vi "Edit Item.vi"(3 "Error in":errorcluster, 5 "Item":u32) -> (0 "Error out":errorcluster)   [LabVIEW 2020]
uses:
  <vilib>/Utility/config.llb/Write Key (String).vi
  <vilib>/Utility/config.llb/NI_LVConfig.lvlib
panel:
  in  "Description":string
  in  "Access Level":enum16{"read-only", "write-only", "read/write"}(ring)
  in  "Data Type":enum16{"Double"}(ring)
  in  "Name":string
  in  "Cancel Button":bool
  in  "OK Button":bool
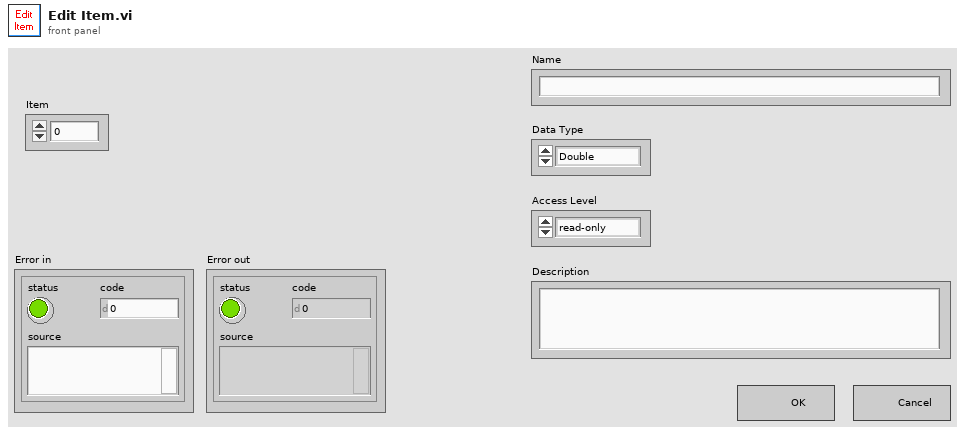
[diagram p1: front panel]
types:
  T1 = cluster{"Name":string, "Data type":u16, "Access level":u16, "Description":string}[]
  T2 = cluster{"Name":string, "Data type":u16, "Access level":u16, "Description":string}
  T3 = typedef "NI_LVConfig.lvlib/Config Data RefNum.ctl" = refnum<k1>
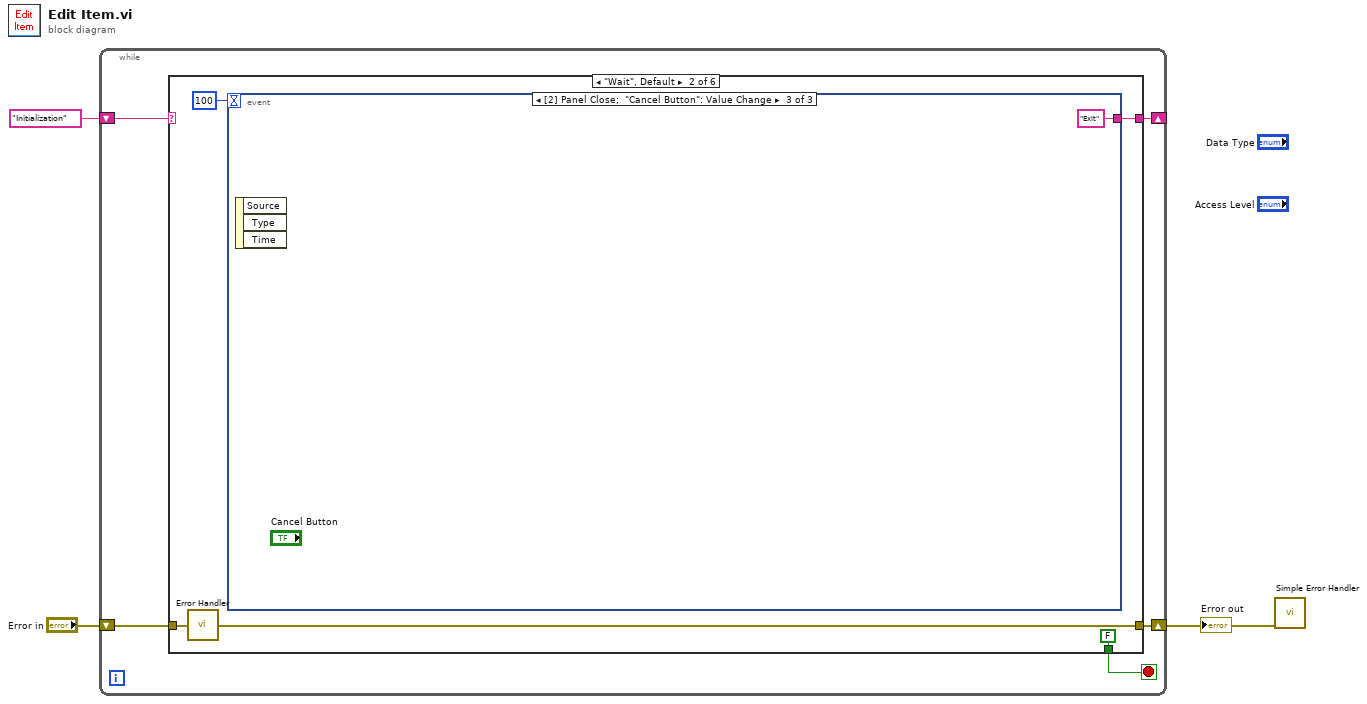
[diagram p0: block diagram]
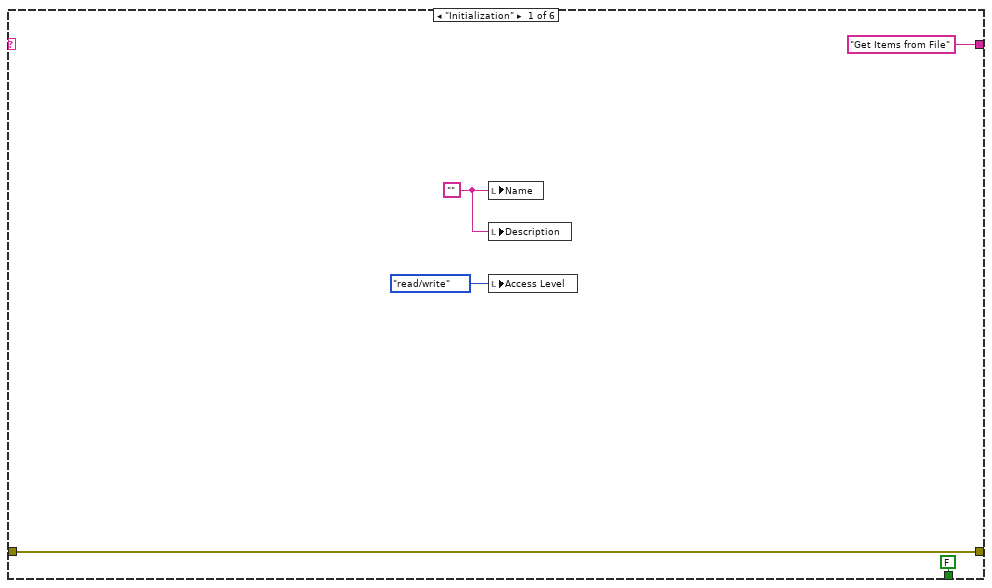
[diagram p2: hidden frame]
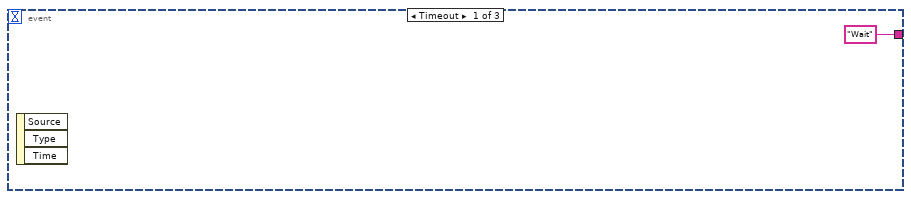
[diagram p3: hidden frame]
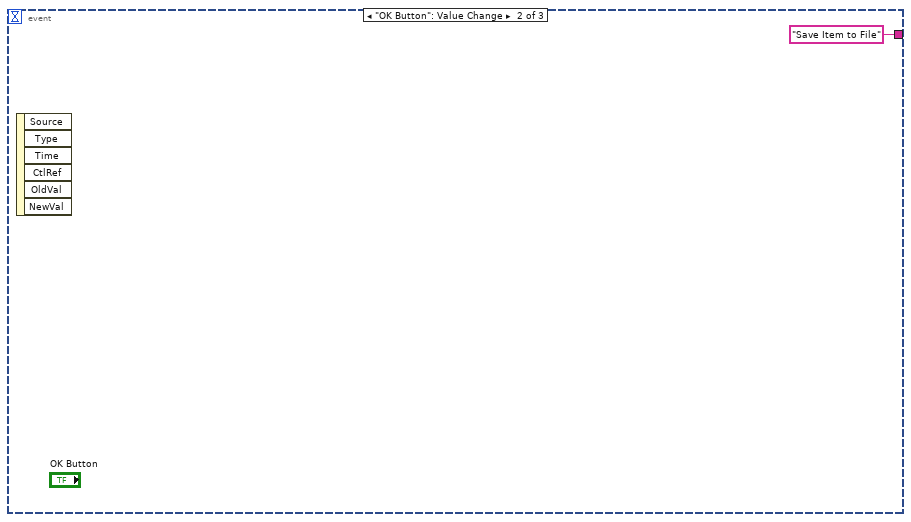
[diagram p4: hidden frame]
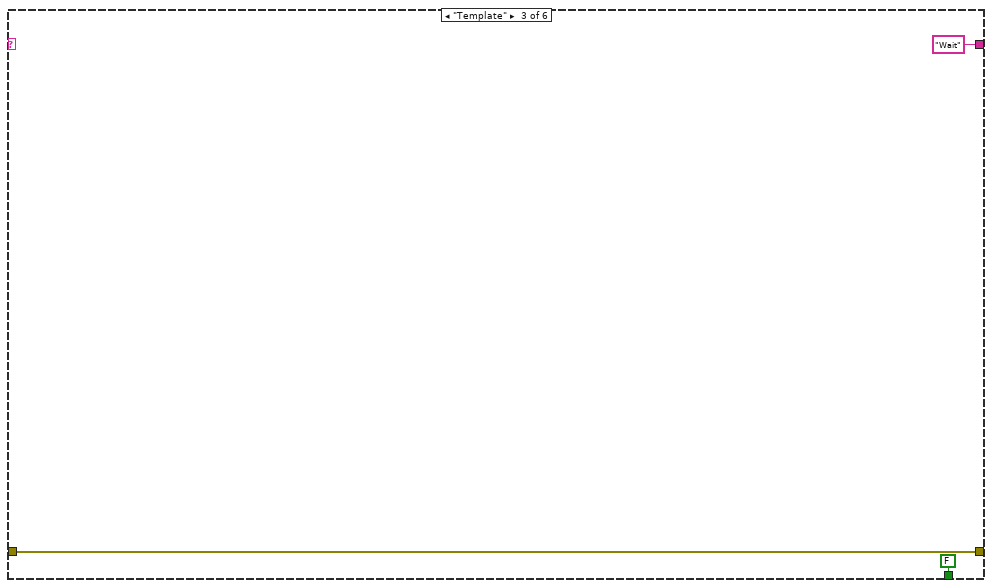
[diagram p5: hidden frame]
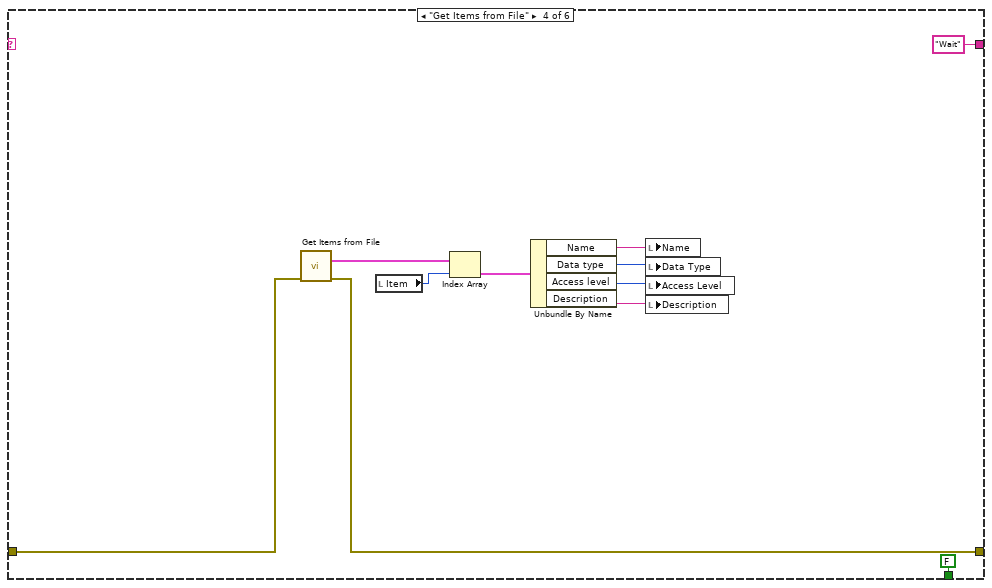
[diagram p6: hidden frame]
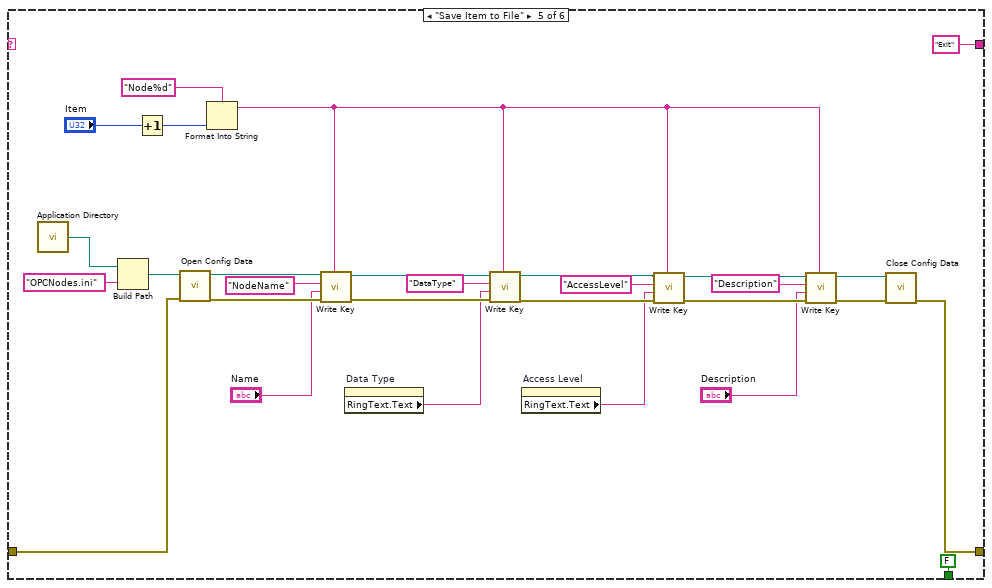
[diagram p7: hidden frame]
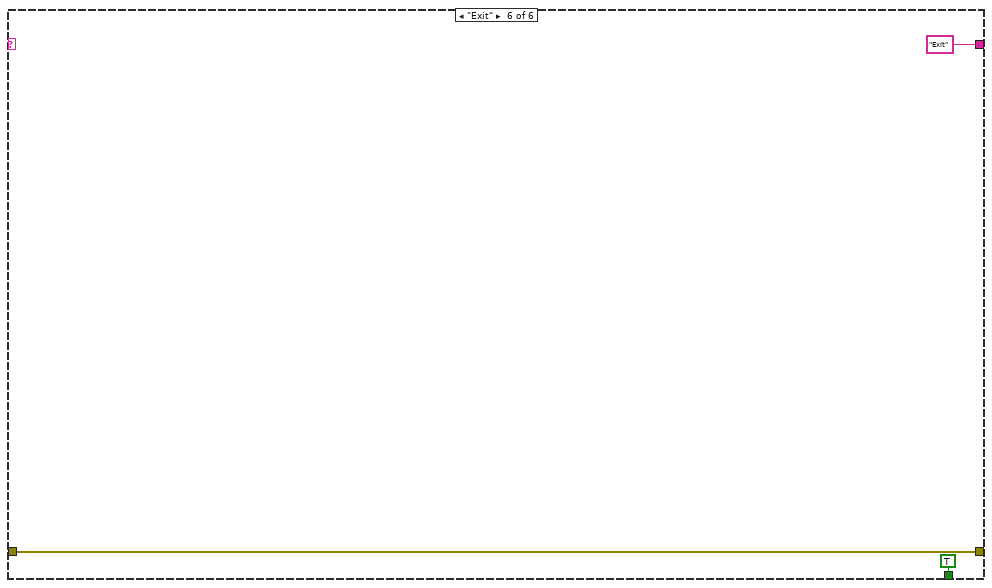
[diagram p8: hidden frame]
diagram:
  n1 = while {
    shift-right: [w7] -> _
    shift-left: "Initialization" -> [w8]
    shift-right: [w4] -> w1
    shift-left: "Error in" -> [w5]
    stop <- w6 stop-if-true
    n2 = case shown="\"Wait\", Default" w8 {
      tunnel: ["Get Items from File" w16 "Wait" "Wait" "Exit" "Exit"] -> w7
      tunnel: [FALSE FALSE FALSE FALSE FALSE TRUE] -> w6
      tunnel: w5 -> [w11 w14 w22 w25 w44 w65]
      tunnel: [w11 w15 w22 w26 w40 w65] -> w4
      frame "Initialization" {
        w9 = ""
        n3 = local write "Name"(w9) -> ()
        n4 = local write "Description"(w9) -> ()
        n5 = local write "Access Level"(enum16{"read-only", "write-only", "read/write"}."read/write" ("Access Level")) -> ()
      }
      frame "Wait", Default {
        n6 = call "Error Handler.vi"("Error in"=w14) -> ("Error out"=w15:errorcluster)
        n7 = event shown="[2] Panel Close;  \"Cancel Button\": Value Change" {
          selector: _ -> [_ _ _]
          dyn-events: _ -> [_ _ _]
          timeout: 100 ("ms") -> [_ _ _]
          tunnel: ["Wait" "Save Item to File" "Exit"] -> w16
          event Timeout {
            n8 = event-data() -> ()  [unwired: 1 in, 3 out]
          }
          event "OK Button": Value Change {
            n9 = event-data() -> ()  [unwired: 1 in, 6 out]
          }
          event Panel Close; "Cancel Button": Value Change {
            n10 = event-data() -> ()  [unwired: 1 in, 3 out]
          }
        }
      }
      frame "Template" {
      }
      frame "Get Items from File" {
        n11 = call "Get Items from File.vi"("Error in"=w25) -> ("Error out"=w26:errorcluster, "Items"=w33:T1)  [unwired: 9 in]
        n12 = local read "Item"() -> (w32:u32)
        n13 = Index Array "Index Array"(array=w33, index=w32) -> (element=w31:T2)
        n14 = Unbundle By Name(w31) -> ("Name"=w30:string, "Data type"=w29:u16, "Access level"=w28:u16, "Description"=w27:string)
        n15 = local write "Name"(w30) -> ()
        n16 = local write "Data Type"(w29) -> ()
        n17 = local write "Access Level"(w28) -> ()
        n18 = local write "Description"(w27) -> ()
      }
      frame "Save Item to File" {
        n19 = call <vilib>:"Application Directory.vi"() -> ("Application Directory"=w62:path)
        n20 = Build Path(base path=w62, name or relative path="OPCNodes.ini") -> (appended path=w60:path)
        n21 = Increment(x="Item") -> (x+1=w37:u32)
        n22 = call <vilib>:"Open Config Data.vi"("error in (no error)"=w44, "configuration file path"=w60) -> ("error out"=w54:errorcluster, "refnum"=w59:T3)  [unwired: 7 in, 1 out]
        n23 = Format Into String(format string="Node%d" ("section"), w37) -> (resulting string=w36:string)  [unwired: 2 in, 1 out]
        n24 = call-poly <vilib>:"Write Key.vi"("section"=w36, "error in (no error)"=w54, "value"="Name", "key"="NodeName", "refnum"=w59) -> ("error out"=w53:errorcluster, "refnum out"=w47:T3)  [unwired: 4 in, 1 out]
        n25 = property on="Data Type" class="Enum (strict)"() -> ("RingText.Text"=w49:string)  [unwired: 2 in, 2 out]
        n26 = call-poly <vilib>:"Write Key.vi"("section"=w36, "error in (no error)"=w53, "value"=w49, "key"="DataType", "refnum"=w47) -> ("error out"=w52:errorcluster, "refnum out"=w46:T3)  [unwired: 4 in, 1 out]
        n27 = property on="Access Level" class="Enum (strict)"() -> ("RingText.Text"=w48:string)  [unwired: 2 in, 2 out]
        n28 = call-poly <vilib>:"Write Key.vi"("section"=w36, "error in (no error)"=w52, "value"=w48, "key"="AccessLevel", "refnum"=w46) -> ("error out"=w51:errorcluster, "refnum out"=w45:T3)  [unwired: 4 in, 1 out]
        n29 = call-poly <vilib>:"Write Key.vi"("section"=w36, "error in (no error)"=w51, "value"="Description", "key"="Description", "refnum"=w45) -> ("error out"=w41:errorcluster, "refnum out"=w42:T3)  [unwired: 4 in, 1 out]
        n30 = call <vilib>:"Close Config Data.vi"("error in (no error)"=w41, "refnum"=w42) -> ("error out"=w40:errorcluster)  [unwired: 8 in, 1 out]
      }
      frame "Exit" {
      }
    }
  }
  "Error out" <- w1
  n31 = call <vilib>:"Simple Error Handler.vi"("error in (no error)"=w1) -> ()  [unwired: 4 in, 5 out]
